vi "irisClose.vi"   [LabVIEW 2017]
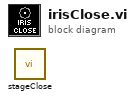
[diagram p0: block diagram]
diagram:
  n1 = call "stageClose.vi"() -> ()  [unwired: 1 out]
